vi "Shooter Control.vi"(11 "Time Delay Milli":u32) -> ()   [LabVIEW 2011]
uses:
  System Set Points and States.vi
  <vilib>/addons/control/pid/pid.llb/PID (DBL).vi
  <vilib>/addons/control/pid/NI_PID_pid.lvlib
panel:
  out "Counter RPM 2":dbl
  out "Stable":bool
  out "RPM Error":cluster{dbl, dbl, dbl[]}(graph)
  out "Output 2":dbl
  out "Output":dbl
  out "Shooter Enabled":bool
  in  "Graph time interval  in seconds":dbl=10.0
  out "Shooter RPM":cluster{dbl, dbl, dbl[]}(graph)
  out "RPM Error":dbl
  out "Encoder Speed":dbl
  out "Encoder Set Speed":dbl
  # "These Work\n0.0045\n0.05\n0.0005"
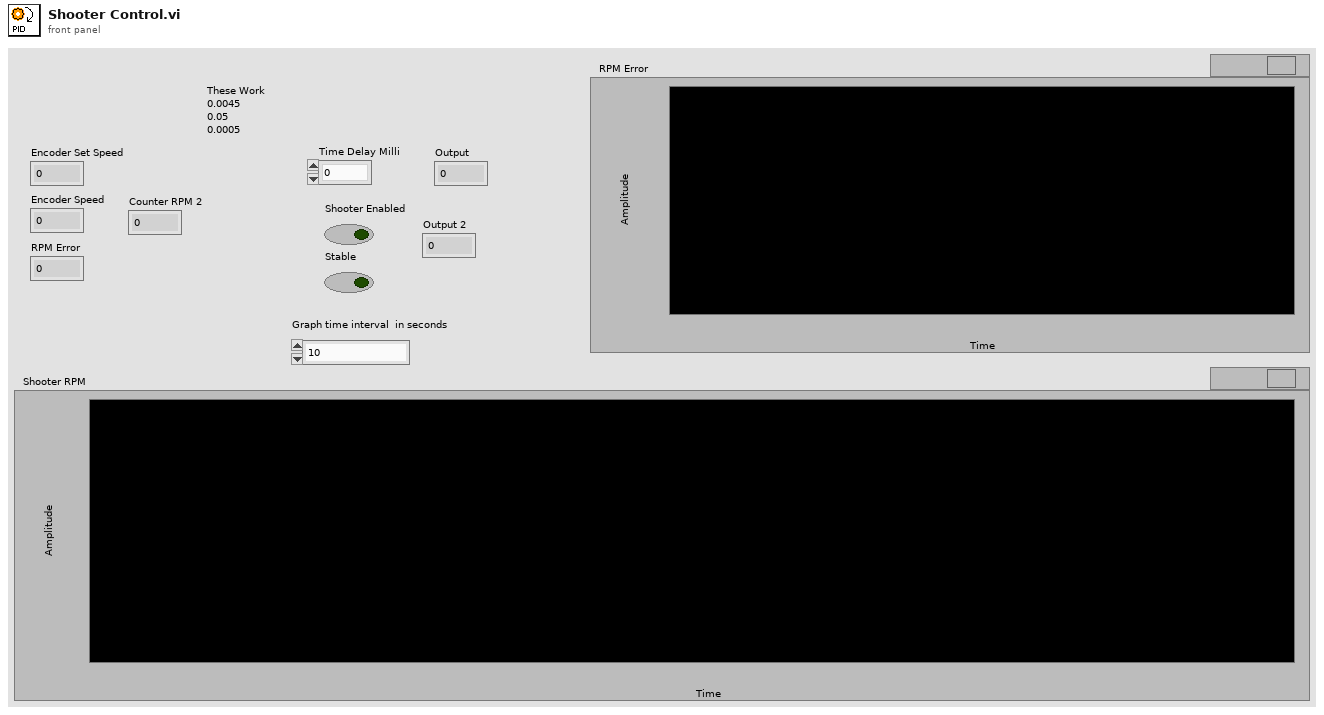
[diagram p1: front panel]
types:
  T1 = cluster{"proportional gain (Kc)":dbl, "integral time (Ti, min)":dbl, "derivative time (Td, min)":dbl}
  T2 = typedef "WPI_CounterDevRef.ctl" = cluster{"DevStatus":errorcluster, "CntIndex":T3}
  T3 = typedef "FPGA_CounterCtrSystemIndex.ctl" = enum8{"Ctr 0", "Ctr 1", "Ctr 2", "Ctr 3", "Ctr 4", "Ctr 5", "Ctr 6", "Ctr 7", "Invalid"}
  T4 = typedef "WPI_EncoderDevRef.ctl" = cluster{"DevStatus":errorcluster, "EncoderIndex":T5, "CounterIndex":T3, "DistancePerCount":dbl, "Decoding Type":T6}
  T5 = typedef "FPGA_EncoderIdx.ctl" = enum8{"Enc 0", "Enc 1", "Enc 2", "Enc 3", "Invalid"}
  T6 = typedef "WPI_EncoderType.ctl" = enum16{"1x", "2x", "4x"}
  T7 = typedef "WPI_MotorControlDeviceRef.ctl" = cluster{"DeviceStatus":errorcluster, "Type":enum16{"PWM", "CAN"}, "PWM":cluster{"Digital Module":T8, "PWM Channel":T9, "DeadBand":T10}, "CAN":cluster{"Device Number":u8, "Control Mode":T11, "Semaphore":T12, "Max Vout":dbl}, "Invert":bool, "TransformRef":T13, "InvTransformRef":T13}
  T8 = typedef "FPGA_TypedefDigitalModule.ctl" = enum16{"Digital Module 1", "Digital Module 2"}
  T9 = typedef "FPGA_DIOPWMChannel.ctl" = enum8{"PWM 1", "PWM 2", "PWM 3", "PWM 4", "PWM 5", "PWM 6", "PWM 7", "PWM 8", "PWM 9", "PWM 10", "Invalid"}
  T10 = typedef "WPI_PWMDeadband.ctl" = cluster{"Name":string, "maxPositivePwm":i32, "minPositivePwm":i32, "centerPwm":i32, "maxNegativePwm":i32, "minNegativePwm":i32, "angularRange":u16}
  T11 = typedef "WPI_CANJaguar_ControlMode.ctl" = enum8{"Percent VBus", "Current", "Speed", "Position", "Voltage"}
  T12 = typedef "Semaphore RefNum" = refnum<k1>
  T13 = typedef "WPI_PWMTransform_ConPane.ctl" = refnum<vi>
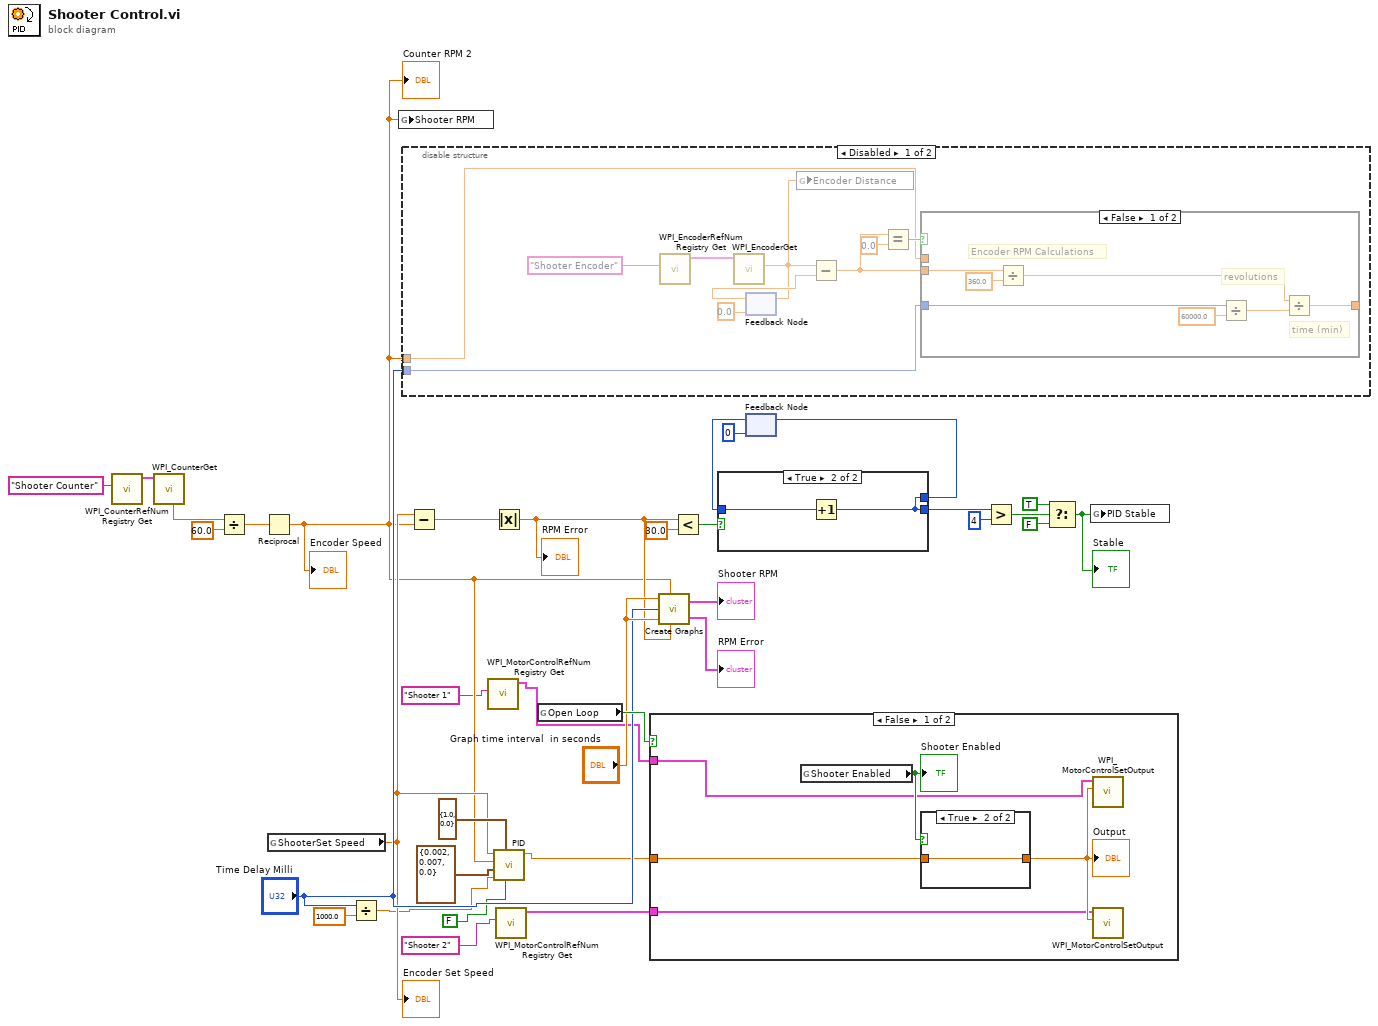
[diagram p0: block diagram]
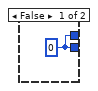
[diagram p2: hidden frame]
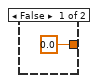
[diagram p5: hidden frame]
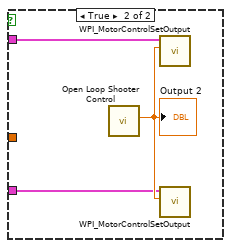
[diagram p6: hidden frame]
diagram:
  n1 = call <vilib>:"WPI_CounterRefNum Registry Get.vi"("refnum name"="Shooter Counter") -> ("CounterDevRef"=w25:T2)  [unwired: 9 in, 1 out]
  n2 = call <vilib>:"WPI_CounterGet.vi"("CounterDevRef in"=w25) -> ("Period (sec)"=w24:dbl)  [unwired: 5 in, 5 out]
  n3 = Divide(x=w24, y=60.0) -> (x/y=w22:dbl)
  n4 = Reciprocal(x=w22) -> (1/x=w8:dbl)
  "Encoder Speed" <- w8
  "Counter RPM 2" <- w8
  n5 = global read "System Set Points and States.vi" "ShooterSet Speed"() -> (w9:dbl)
  "Encoder Set Speed" <- w9
  n6 = Divide(x="Time Delay Milli", y=1000.0) -> (x/y=w7:dbl)
  n7 = global write "System Set Points and States.vi" "Shooter RPM"(w8) -> ()
  n8 = disable-structure shown="Disabled" {
    disable-tunnel: "Time Delay Milli" -> [w37 _]
    disable-tunnel: w8 -> [w36 _]
    frame Disabled {
      n9 = call <vilib>:"WPI_EncoderRefNum Registry Get.vi"("refnum name"="Shooter Encoder") -> ("EncoderDevRef"=w40:T4)  [unwired: 9 in, 1 out]
      n10 = call <vilib>:"WPI_EncoderGet.vi"("EncoderDevRef"=w40) -> ("Distance"=w38:dbl)  [unwired: 5 in, 5 out]
      n11 = feedback #1(0.0) -> (w45:dbl)
      n12 = feedback-in #1(w38) -> ()
      n13 = global write "System Set Points and States.vi" "Encoder Distance"(w38) -> ()
      n14 = Subtract(x=w38, y=w45) -> (x-y=w39:dbl)
      n15 = Equal?(x=w39, y=0.0) -> (x = y?=w42:bool)
      n16 = case shown="False" w42 {
        tunnel: [w52 w53] -> _
        tunnel: w39 -> [w51 _]
        tunnel: w37 -> [w49 _]
        tunnel: w36 -> [_ w53]
        frame False {
          # "time (min)"
          # "revolutions"
          # "Encoder RPM Calculations"
          n17 = Divide(x=w51, y=360.0) -> (x/y=w50:dbl)
          n18 = Divide(x=w49, y=60000.0) -> (x/y=w47:dbl)
          n19 = Divide(x=w50, y=w47) -> (x/y=w52:dbl)
        }
        frame True {
        }
      }
    }
    frame Enabled {
    }
  }
  n20 = Subtract(x=w9, y=w8) -> (x-y=w28:dbl)
  n21 = call <vilib>:"WPI_MotorControlRefNum Registry Get.vi"("refnum name"="Shooter 1") -> ("MotorControlDevRef"=w4:T7)  [unwired: 9 in, 1 out]
  n22 = Absolute Value(x=w28) -> (abs(x)=w27:dbl)
  "RPM Error" <- w27
  n23 = call-poly <vilib>:"PID.vi"("reinitialize? (F)"=FALSE, "output range"=cluster{"output high":dbl, "output low":dbl} {"output high"=1.0, "output low"=0.0}, "dt (s)"=w7, "PID gains"=T1 {"proportional gain (Kc)"=0.002, "integral time (Ti, min)"=0.007, "derivative time (Td, min)"=0.0}, "process variable"=w8, "setpoint"=w9) -> ("output"=w5:dbl)  [unwired: 4 in, 1 out]
  n24 = call <vilib>:"WPI_MotorControlRefNum Registry Get.vi"("refnum name"="Shooter 2") -> ("MotorControlDevRef"=w2:T7)  [unwired: 9 in, 1 out]
  n25 = global read "System Set Points and States.vi" "Open Loop"() -> (w35:bool)
  n26 = case shown="False" w35 {
    tunnel: w2 -> [w56 w61]
    tunnel: w4 -> [w55 w62]
    tunnel: w5 -> [w54 _]
    frame False {
      n27 = global read "System Set Points and States.vi" "Shooter Enabled"() -> (w58:bool)
      "Shooter Enabled" <- w58
      n28 = case shown="True" w58 {
        tunnel: [0.0 ("output") w60] -> w57
        tunnel: w54 -> [_ w60]
        frame False {
        }
        frame True {
        }
      }
      "Output" <- w57
      n29 = call <vilib>:"WPI_MotorControlSetOutput.vi"("Output"=w57, "MotorControlDevRef"=w55) -> ()  [unwired: 8 in, 2 out]
      n30 = call <vilib>:"WPI_MotorControlSetOutput.vi"("Output"=w57, "MotorControlDevRef"=w56) -> ()  [unwired: 8 in, 2 out]
    }
    frame True {
      n31 = call "Open Loop Shooter Control.vi"() -> ("Open Loop PWM"=w63:dbl)  [unwired: 11 in]
      "Output 2" <- w63
      n32 = call <vilib>:"WPI_MotorControlSetOutput.vi"("Output"=w63, "MotorControlDevRef"=w62) -> ()  [unwired: 8 in, 2 out]
      n33 = call <vilib>:"WPI_MotorControlSetOutput.vi"("Output"=w63, "MotorControlDevRef"=w61) -> ()  [unwired: 8 in, 2 out]
    }
  }
  n34 = call "Create Graphs.vi"("Speed Graph Time"="Graph time interval  in seconds", "Speed"=w8, "Time Delay"="Time Delay Milli", "Error Graph Time"="Graph time interval  in seconds", "Error"=w27) -> ("Speed"=→"Shooter RPM":cluster{dbl, dbl, dbl[]}, "Error"=→"RPM Error":cluster{dbl, dbl, dbl[]})
  n35 = Less?(x=w27, y=30.0) -> (x < y?=w21:bool)
  n36 = feedback #2(0) -> (w20:i32)
  n37 = case shown="True" w21 {
    tunnel: [w64 w65] -> w19
    tunnel: w20 -> [_ w66]
    tunnel: [w64 w65] -> w16
    frame False {
      w64 = 0
    }
    frame True {
      n38 = Increment(x=w66) -> (x+1=w65:i32)
    }
  }
  n39 = feedback-in #2(w19) -> ()
  n40 = Greater?(x=w16, y=4) -> (0:w17:bool)
  n41 = Select(t=TRUE, s=w17, f=FALSE) -> (s? t:f=w12:bool)
  "Stable" <- w12
  n42 = global write "System Set Points and States.vi" "PID Stable"(w12) -> ()
